vi "Measurement UI.vi"() -> ()   [LabVIEW 2021, in "Line Regulation_PMIC.lvlib"]
uses:
  Line Regulation_PMIC.lvlib
panel:
  in  "MeasGraphs":T1(tab)
  out "LineRegulationGraph(V/V)":T2(graph)
  out "LineRegulationGraph(%)":T3(graph)
  out "Load voltage deviation":dbl[](array[numeric])
  out "Load voltages":dbl[](array[numeric])
  out "Source voltages":dbl[](array[numeric])
  in  "Source resource name":string caption="RESOURCE NAME"
  in  "Load resource name":string caption="RESOURCE NAME"
  out "Measured current limit":dbl format="%#_6p"
  out "Measured voltage level":dbl format="%#_6p"
  out "Status":string
  in  "ELOADResourceName":refnum<k15> caption="RESOURCE NAME"
  in  "PPSResourceName":refnum<k15> caption="RESOURCE NAME"
  in  "Source sweep type":string(combo)="Logarithmic" caption="SWEEP TYPE"
  in  "DUT setup time":dbl=1.0 caption="DUT SETUP TIME" format="%#_6ps"
  in  "Source stop voltage":dbl=20.0 caption="STOP VOLTAGE" format="%#_6pV"
  in  "Source start voltage":dbl=6.0 caption="START VOLTAGE" format="%#_6pV"
  in  "Source voltage sweep points/points per decade":i32=10 caption="PTS/PTS PER DECADE"
  in  "Aperture time":dbl=0.005 caption="APERTURE TIME" format="%#_6ps"
  in  "Source delay":dbl=0.005 caption="SOURCE DELAY" format="%#_6ps"
  in  "Load current level":dbl=1.0 caption="CURRENT  LEVEL" format="%#_6pA"
  in  "Load voltage limit range":dbl=6.0 caption="VOLTAGE LIMIT RANGE" format="%#_6pV"
  in  "Source current limit":dbl=25.0 caption="CURRENT LIMIT" format="%#_6pA"
  in  "Source maximum power":dbl=300.0 caption="MAXIMUM POWER" format="%#_6pW"
  in  "Load configuration":string="Load configuration"
  in  "Source configuration":string="Source configuration"
  in  "Measurement settings":string="Measurement settings"
  in  "Nominal output voltage":dbl=3.3 caption="NOMINAL OUTPUT VOLTAGE" format="%#_6pV"
  in  "Mode of operation":T4(ring)=enum."Perform measurement" caption="MODE OF OPERATION"
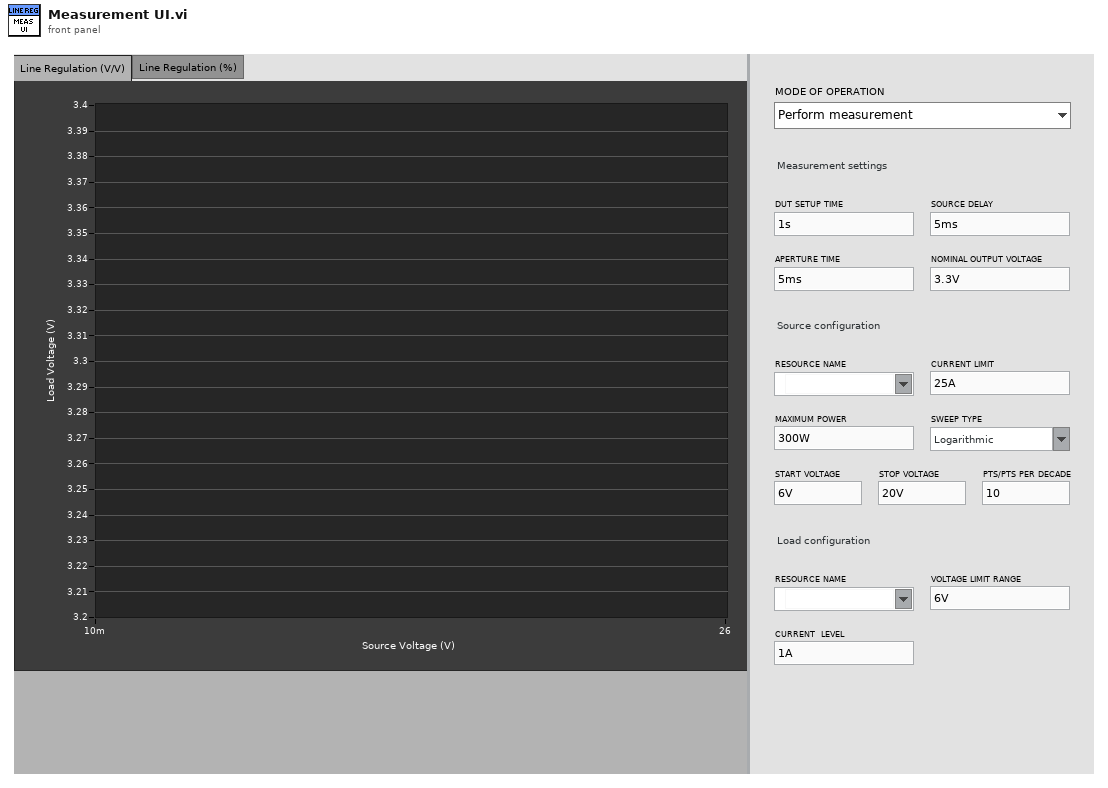
[diagram p1: front panel]
types:
  T1 = enum32{"Line Regulation (V/V)", "Line Regulation (%)", "Hidden Controls"}
  T2 = cluster{"Source voltages":dbl[], "Load voltages":dbl[]}
  T3 = cluster{"Source voltages":dbl[], "Load voltage deviation":dbl[]}
  T4 = enum32{"Power on the DUT", "Perform measurement", "Power off the DUT"}
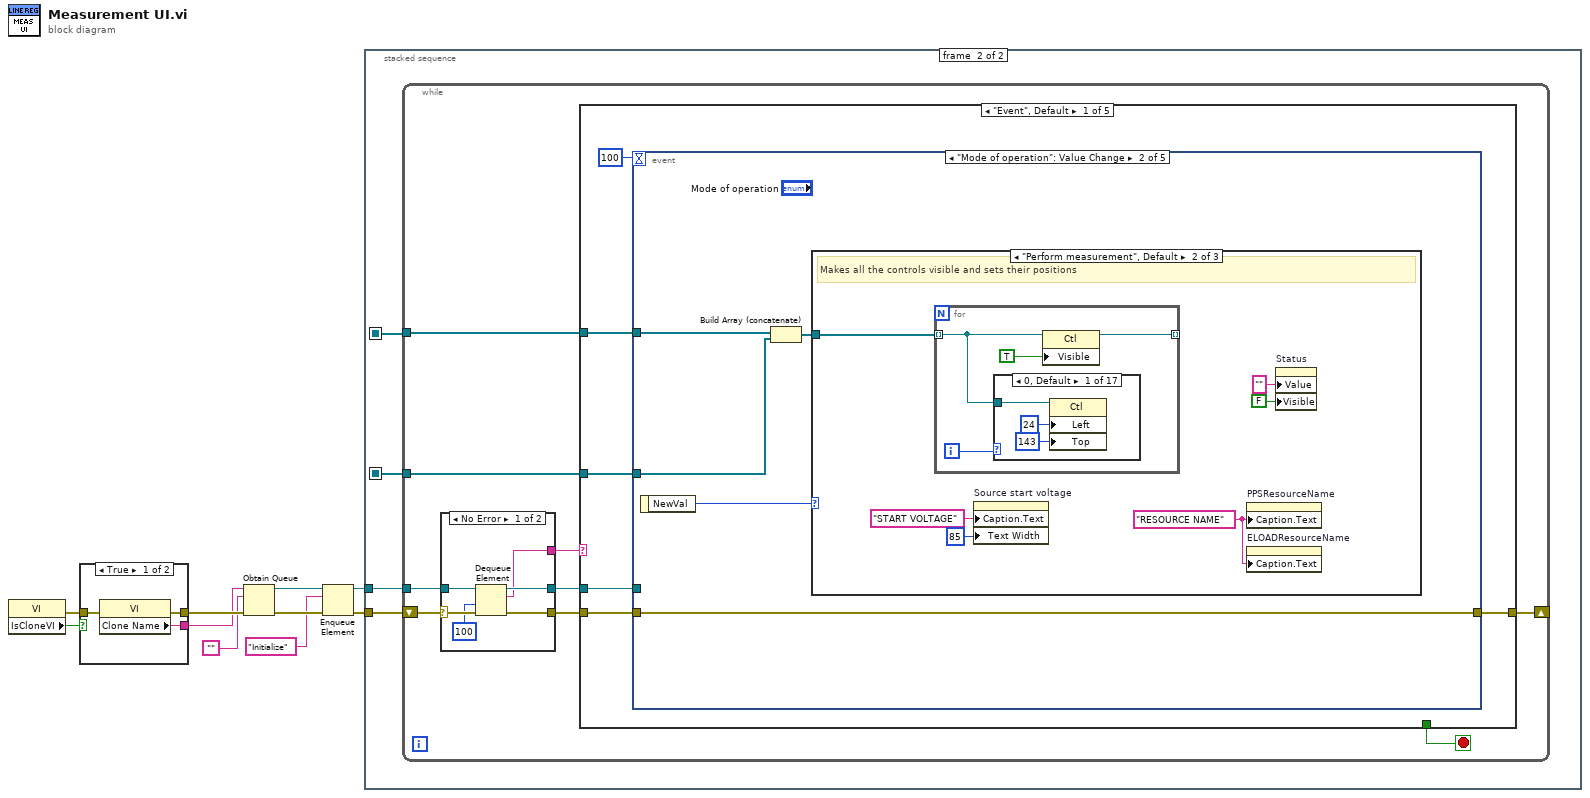
[diagram p0: block diagram]
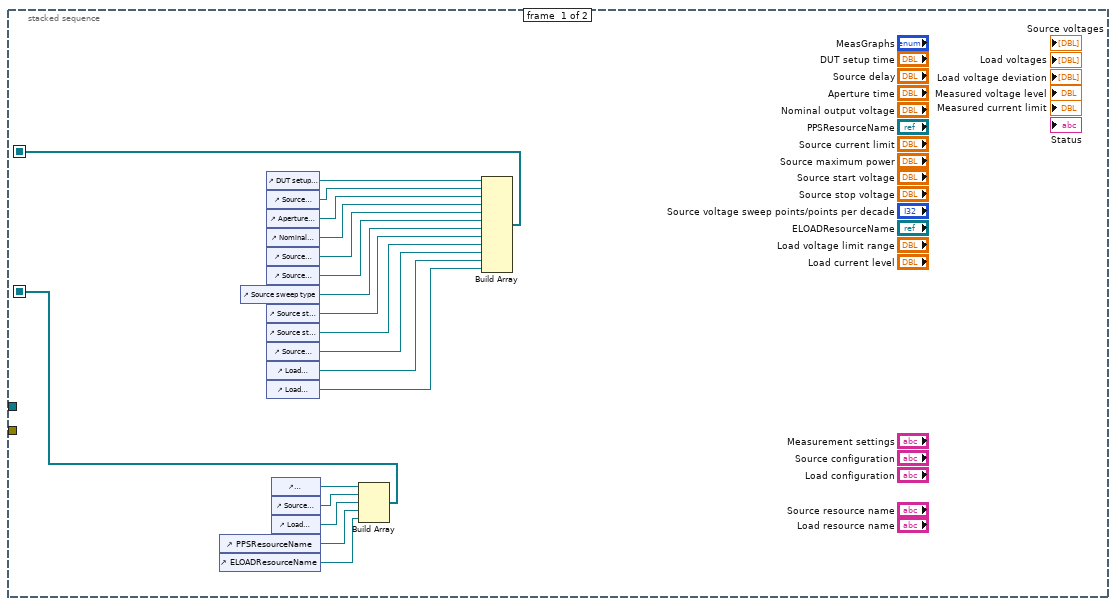
[diagram p2: hidden frame]
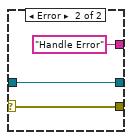
[diagram p3: hidden frame]
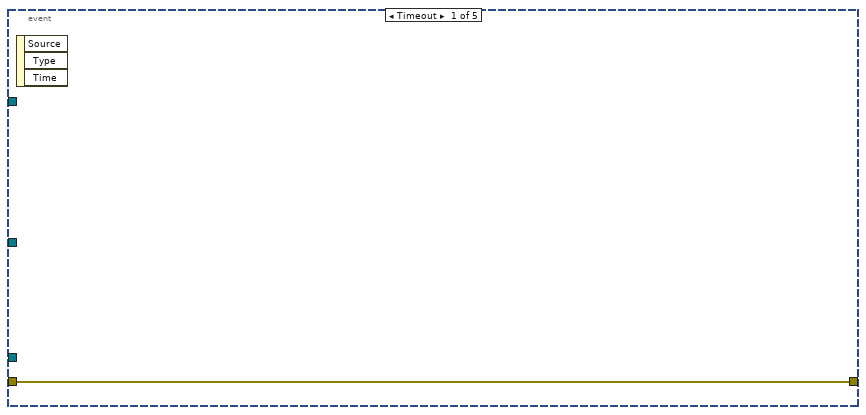
[diagram p4: hidden frame]
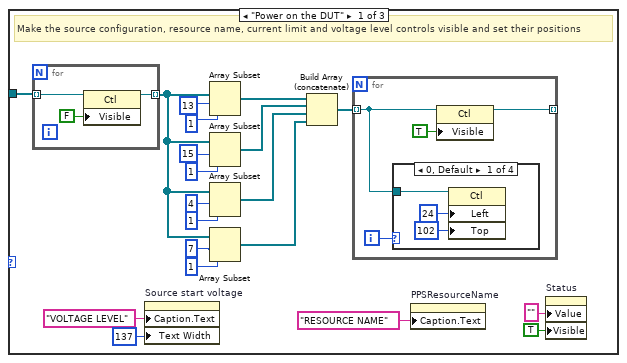
[diagram p5: hidden frame]
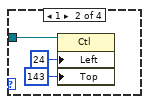
[diagram p6: hidden frame]
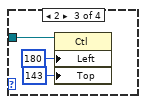
[diagram p7: hidden frame]
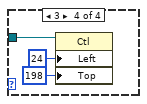
[diagram p8: hidden frame]
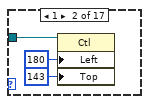
[diagram p9: hidden frame]
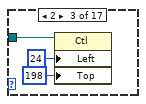
[diagram p10: hidden frame]
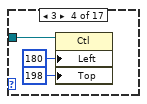
[diagram p11: hidden frame]
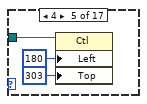
[diagram p12: hidden frame]
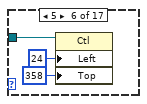
[diagram p13: hidden frame]
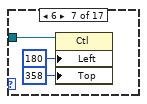
[diagram p14: hidden frame]
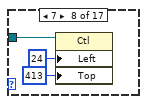
[diagram p15: hidden frame]
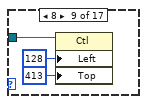
[diagram p16: hidden frame]
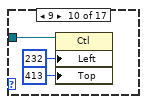
[diagram p17: hidden frame]
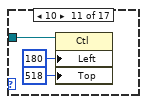
[diagram p18: hidden frame]
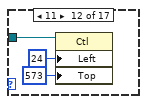
[diagram p19: hidden frame]
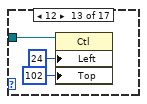
[diagram p20: hidden frame]
diagram:
  n1 = property class="VI"() -> (error out=w1:errorcluster, "IsCloneVI"=w2:bool)  [unwired: 2 in, 1 out]
  n2 = case shown="True" w2 {
    tunnel: [w13 w16] -> w10
    tunnel: [w12 w15] -> w9
    tunnel: w1 -> [w11 w14]
    frame True {
      n3 = property class="VI"(error in=w11) -> (error out=w13:errorcluster, "Clone Name"=w12:string)  [unwired: 1 in, 1 out]
    }
    frame False {
      n4 = property class="VI"(error in=w14) -> (error out=w16:errorcluster, "Name"=w15:string)  [unwired: 1 in, 1 out]
    }
  }
  n5 = Obtain Queue(name (unnamed)=w9, element data type="", error in (no error)=w10) -> (queue out=w6:refnum<queue>, error out=w8:errorcluster)  [unwired: 2 in, 1 out]
  n6 = Enqueue Element(queue=w6, element="Initialize", error in (no error)=w8) -> (queue out=w5:refnum<queue>, error out=w7:errorcluster)  [unwired: 1 in, 1 out]
  n7 = stacked-sequence {
    seq-local: [w18 _] -> [_ w37]
    seq-local: [w17 _] -> [_ w36]
    tunnel: w7 -> [_ w39]
    tunnel: w5 -> [_ w38]
    frame #0 {
      n8 = control-ref of="PPSResourceName"() -> (w21:refnum<vi>)
      n9 = control-ref of="ELOADResourceName"() -> (w20:refnum<vi>)
      n10 = control-ref of="Source sweep type"() -> (w19:refnum<vi>)
      n11 = control-ref of="DUT setup time"() -> (w35:refnum<vi>)
      n12 = control-ref of="Source delay"() -> (w34:refnum<vi>)
      n13 = control-ref of="Aperture time"() -> (w33:refnum<vi>)
      n14 = control-ref of="Nominal output voltage"() -> (w25:refnum<vi>)
      n15 = control-ref of="Source current limit"() -> (w32:refnum<vi>)
      n16 = control-ref of="Source maximum power"() -> (w31:refnum<vi>)
      n17 = control-ref of="Source start voltage"() -> (w30:refnum<vi>)
      n18 = control-ref of="Source stop voltage"() -> (w29:refnum<vi>)
      n19 = control-ref of="Source voltage sweep points/points per decade"() -> (w28:refnum<vi>)
      n20 = control-ref of="Load voltage limit range"() -> (w27:refnum<vi>)
      n21 = control-ref of="Load current level"() -> (w26:refnum<vi>)
      n22 = control-ref of="Measurement settings"() -> (w24:refnum<vi>)
      n23 = control-ref of="Source configuration"() -> (w22:refnum<vi>)
      n24 = control-ref of="Load configuration"() -> (w23:refnum<vi>)
      n25 = Build Array(w24, w22, w23, w21, w20) -> (w17:refnum<vi>[])
      n26 = Build Array(w35, w34, w33, w25, w32, w31, w19, w30, w29, w28, w27, w26) -> (w18:refnum<vi>[])
    }
    frame #1 {
      n27 = while {
        shift-right: [w43] -> _
        shift-left: w39 -> [w48]
        tunnel: w38 -> [w46]
        tunnel: w37 -> [w41]
        tunnel: w36 -> [w40]
        stop <- w42 stop-if-true
        n28 = case shown="No Error" w48 {
          selector: w48 -> [w54 w57]
          tunnel: [w53 w57] -> w47
          tunnel: w46 -> [w52 w56]
          tunnel: [w51 w56] -> w45
          tunnel: [w50 "Handle Error"] -> w44
          frame No Error {
            n29 = Dequeue Element(queue=w52, timeout in ms (-1)=100, error in (no error)=w54) -> (queue out=w51:refnum<queue>, element=w50:string, error out=w53:errorcluster)  [unwired: 1 out]
          }
          frame Error {
          }
        }
        n30 = case shown="\"Event\", Default" w44 {
          tunnel: w47 -> [w62 w206 w221 w235 w236]
          tunnel: w45 -> [w60 _ _ w233 _]
          tunnel: [w63 w206 w221 w227 w236] -> w43
          tunnel: [_ _ _ TRUE _] -> w42
          tunnel: w41 -> [w59 _ _ w226 _]
          tunnel: w40 -> [w58 _ _ w225 _]
          frame "Event", Default {
            n31 = event shown="[1] \"Mode of operation\": Value Change" {
              selector: _ -> [_ _ _ _ _]
              dyn-events: _ -> [_ _ _ _ _]
              timeout: 100 -> [_ _ _ _ _]
              tunnel: [w64 w65 w192 w194 w198] -> w63
              tunnel: w62 -> [w64 w65 w192 w194 w199]
              tunnel: w60 -> [_ _ _ _ w197]
              tunnel: w59 -> [_ w66 _ _ _]
              tunnel: w58 -> [_ w68 _ _ _]
              event Timeout {
                n32 = event-data() -> ()  [unwired: 1 in, 3 out]
              }
              event "Mode of operation": Value Change {
                n33 = event-data() -> ("NewVal"=w69:T4)  [unwired: 1 in]
                n34 = Build Array (concatenate)(w66, w68) -> (w67:refnum<vi>[])
                n35 = case shown="\"Perform measurement\", Default" w69 {
                  tunnel: w67 -> [w81 w114 w175]
                  frame "Power on the DUT" {
                    # "Make the source configuration, resource name, current limit and voltage level controls visible and set their positions"
                    n36 = for {
                      tunnel: w81 -> [w92] mode=indexing
                      tunnel: [w90] -> w78 mode=indexing
                      n37 = property class="Ctl"(reference=w92, "Visible"=FALSE) -> (reference out=w90:refnum<vi>)  [unwired: 1 in, 1 out]
                    }
                    n38 = property on="Source start voltage" class="DigNum (strict)"("Caption.Text"="VOLTAGE LEVEL", "Text Width"=u32 137) -> ()  [unwired: 2 in, 2 out]
                    n39 = Array Subset(array=w78, index=13 ("length"), length=1 ("index")) -> (w80:refnum<vi>[])
                    n40 = Array Subset(array=w78, index=15 ("length"), length=1 ("index")) -> (w79:refnum<vi>[])
                    n41 = Array Subset(array=w78, index=4 ("length"), length=1 ("index")) -> (w77:refnum<vi>[])
                    n42 = Array Subset(array=w78, index=7 ("length"), length=1 ("index")) -> (w75:refnum<vi>[])
                    n43 = Build Array (concatenate)(w80, w79, w77, w75) -> (w76:refnum<vi>[])
                    n44 = for {
                      tunnel: [w95] -> _ mode=indexing
                      tunnel: w76 -> [w93] mode=indexing
                      i -> [w94]
                      n45 = case shown="0, Default" w94 {
                        tunnel: w93 -> [w99 w102 w105 w108]
                        frame 0, Default {
                          n46 = property class="Ctl"(reference=w99, "Left"=24 ("Position:Left"), "Top"=102 ("Position:Top")) -> ()  [unwired: 1 in, 2 out]
                        }
                        frame 1 {
                          n47 = property class="Ctl"(reference=w102, "Left"=24 ("Position:Left"), "Top"=143 ("Position:Top")) -> ()  [unwired: 1 in, 2 out]
                        }
                        frame 2 {
                          n48 = property class="Ctl"(reference=w105, "Left"=180 ("Position:Left"), "Top"=143 ("Position:Top")) -> ()  [unwired: 1 in, 2 out]
                        }
                        frame 3 {
                          n49 = property class="Ctl"(reference=w108, "Left"=24 ("Position:Left"), "Top"=198 ("Position:Top")) -> ()  [unwired: 1 in, 2 out]
                        }
                      }
                      n50 = property class="Ctl"(reference=w93, "Visible"=TRUE) -> (reference out=w95:refnum<vi>)  [unwired: 1 in, 1 out]
                    }
                    n51 = property on="PPSResourceName" class="IVIName"("Caption.Text"="RESOURCE NAME") -> ()  [unwired: 2 in, 2 out]
                    n52 = property on="Status" class="Str"("Value"="" ("Operation"), "Visible"=TRUE) -> ()  [unwired: 2 in, 2 out]
                  }
                  frame "Perform measurement", Default {
                    w112 = "RESOURCE NAME" ("Caption.Text")
                    # "Makes all the controls visible and sets their positions"
                    n53 = for {
                      tunnel: w114 -> [w115] mode=indexing
                      tunnel: [w117] -> _ mode=indexing
                      i -> [w116]
                      n54 = case shown="0, Default" w116 {
                        tunnel: w115 -> [w121 w124 w127 w130 w133 w136 w139 w142 w145 w148 w151 w154 w157 w160 w163 w166 w169]
                        frame 0, Default {
                          n55 = property class="Ctl"(reference=w121, "Left"=24 ("Position:Left"), "Top"=143 ("Position:Top")) -> ()  [unwired: 1 in, 2 out]
                        }
                        frame 1 {
                          n56 = property class="Ctl"(reference=w124, "Left"=180 ("Position:Left"), "Top"=143 ("Position:Top")) -> ()  [unwired: 1 in, 2 out]
                        }
                        frame 2 {
                          n57 = property class="Ctl"(reference=w127, "Left"=24 ("Position:Left"), "Top"=198 ("Position:Top")) -> ()  [unwired: 1 in, 2 out]
                        }
                        frame 3 {
                          n58 = property class="Ctl"(reference=w130, "Left"=180 ("Position:Left"), "Top"=198 ("Position:Top")) -> ()  [unwired: 1 in, 2 out]
                        }
                        frame 4 {
                          n59 = property class="Ctl"(reference=w133, "Left"=180 ("Position:Left"), "Top"=303 ("Position:Top")) -> ()  [unwired: 1 in, 2 out]
                        }
                        frame 5 {
                          n60 = property class="Ctl"(reference=w136, "Left"=24 ("Position:Left"), "Top"=358 ("Position:Top")) -> ()  [unwired: 1 in, 2 out]
                        }
                        frame 6 {
                          n61 = property class="Ctl"(reference=w139, "Left"=180 ("Position:Left"), "Top"=358 ("Position:Top")) -> ()  [unwired: 1 in, 2 out]
                        }
                        frame 7 {
                          n62 = property class="Ctl"(reference=w142, "Left"=24 ("Position:Left"), "Top"=413 ("Position:Top")) -> ()  [unwired: 1 in, 2 out]
                        }
                        frame 8 {
                          n63 = property class="Ctl"(reference=w145, "Left"=128 ("Position:Left"), "Top"=413 ("Position:Top")) -> ()  [unwired: 1 in, 2 out]
                        }
                        frame 9 {
                          n64 = property class="Ctl"(reference=w148, "Left"=232 ("Position:Left"), "Top"=413 ("Position:Top")) -> ()  [unwired: 1 in, 2 out]
                        }
                        frame 10 {
                          n65 = property class="Ctl"(reference=w151, "Left"=180 ("Position:Left"), "Top"=518 ("Position:Top")) -> ()  [unwired: 1 in, 2 out]
                        }
                        frame 11 {
                          n66 = property class="Ctl"(reference=w154, "Left"=24 ("Position:Left"), "Top"=573 ("Position:Top")) -> ()  [unwired: 1 in, 2 out]
                        }
                        frame 12 {
                          n67 = property class="Ctl"(reference=w157, "Left"=24 ("Position:Left"), "Top"=102 ("Position:Top")) -> ()  [unwired: 1 in, 2 out]
                        }
                        frame 13 {
                          n68 = property class="Ctl"(reference=w160, "Left"=24 ("Position:Left"), "Top"=262 ("Position:Top")) -> ()  [unwired: 1 in, 2 out]
                        }
                        frame 14 {
                          n69 = property class="Ctl"(reference=w163, "Left"=24 ("Position:Left"), "Top"=477 ("Position:Top")) -> ()  [unwired: 1 in, 2 out]
                        }
                        frame 15 {
                          n70 = property class="Ctl"(reference=w166, "Left"=24 ("Position:Left"), "Top"=303 ("Position:Top")) -> ()  [unwired: 1 in, 2 out]
                        }
                        frame 16 {
                          n71 = property class="Ctl"(reference=w169, "Left"=24 ("Position:Left"), "Top"=518 ("Position:Top")) -> ()  [unwired: 1 in, 2 out]
                        }
                      }
                      n72 = property class="Ctl"(reference=w115, "Visible"=TRUE) -> (reference out=w117:refnum<vi>)  [unwired: 1 in, 1 out]
                    }
                    n73 = property on="Source start voltage" class="DigNum (strict)"("Caption.Text"="START VOLTAGE", "Text Width"=u32 85) -> ()  [unwired: 2 in, 2 out]
                    n74 = property on="PPSResourceName" class="IVIName"("Caption.Text"=w112) -> ()  [unwired: 2 in, 2 out]
                    n75 = property on="ELOADResourceName" class="IVIName"("Caption.Text"=w112) -> ()  [unwired: 2 in, 2 out]
                    n76 = property on="Status" class="Str"("Value"="" ("Status"), "Visible"=FALSE) -> ()  [unwired: 2 in, 2 out]
                  }
                  frame "Power off the DUT" {
                    # "Makes only the Source and Load Resource Name controls visible and sets their positions"
                    n77 = for {
                      tunnel: w175 -> [w180] mode=indexing
                      tunnel: [w179] -> w174 mode=indexing
                      n78 = property class="Ctl"(reference=w180, "Visible"=FALSE) -> (reference out=w179:refnum<vi>)  [unwired: 1 in, 1 out]
                    }
                    n79 = Array Subset(array=w174, index=15 ("length"), length=2 ("index")) -> (w176:refnum<vi>[])
                    n80 = property on="PPSResourceName" class="IVIName"("Caption.Text"="SOURCE RESOURCE NAME") -> ()  [unwired: 2 in, 2 out]
                    n81 = property on="ELOADResourceName" class="IVIName"("Caption.Text"="LOAD RESOURCE NAME") -> ()  [unwired: 2 in, 2 out]
                    n82 = for {
                      tunnel: w176 -> [w182] mode=indexing
                      tunnel: [w184] -> _ mode=indexing
                      i -> [w183]
                      n83 = case shown="0, Default" w183 {
                        tunnel: w182 -> [w188 w191]
                        frame 0, Default {
                          n84 = property class="Ctl"(reference=w188, "Left"=24 ("Position:Left"), "Top"=102 ("Position:Top")) -> ()  [unwired: 1 in, 2 out]
                        }
                        frame 1 {
                          n85 = property class="Ctl"(reference=w191, "Left"=24 ("Position:Left"), "Top"=157 ("Position:Top")) -> ()  [unwired: 1 in, 2 out]
                        }
                      }
                      n86 = property class="Ctl"(reference=w182, "Visible"=TRUE) -> (reference out=w184:refnum<vi>)  [unwired: 1 in, 1 out]
                    }
                    n87 = property on="Status" class="Str"("Value"="" ("Operation"), "Visible"=TRUE) -> ()  [unwired: 2 in, 2 out]
                  }
                }
              }
              event "PPSResourceName": Value Change {
                n88 = event-data() -> ()  [unwired: 1 in, 1 out]
                n89 = property on="PPSResourceName" class="IVIName"() -> ("Value"=w193:refnum<k15>)  [unwired: 2 in, 2 out]
                n90 = property on="Source resource name" class="Str"("Value"=w193) -> ()  [unwired: 2 in, 2 out]
              }
              event "ELOADResourceName": Value Change {
                n91 = event-data() -> ()  [unwired: 1 in, 1 out]
                n92 = property on="ELOADResourceName" class="IVIName"() -> ("Value"=w195:refnum<k15>)  [unwired: 2 in, 2 out]
                n93 = property on="Load resource name" class="Str"("Value"=w195) -> ()  [unwired: 2 in, 2 out]
              }
              event Panel Close? {
                n94 = event-data() -> ()  [unwired: 1 in, 1 out]
                n95 = Enqueue Element(queue=w197, element="Exit", error in (no error)=w199) -> (error out=w198:errorcluster)  [unwired: 1 in, 2 out]
                n96 = event-data("Discard?"=TRUE) -> ()  [unwired: 1 in, 1 out]
              }
            }
          }
          frame "Initialize" {
            w205 = "<Select Device>"
            n97 = control-ref of="LineRegulationGraph(V/V)"() -> (w204:refnum<vi>)
            n98 = control-ref of="LineRegulationGraph(%)"() -> (w203:refnum<vi>)
            n99 = Build Array(w204, w203) -> (w202:refnum<vi>[])
            n100 = for {
              tunnel: w202 -> [w207] mode=indexing
              n101 = property class="XYGraph (strict)"(reference=w207, "ActPaletteTool"=2 ("Palette:Active Tool")) -> ()  [unwired: 1 in, 2 out]
            }
            n102 = property on="PPSResourceName" class="IVIName"("Value"=w205) -> ()  [unwired: 2 in, 2 out]
            n103 = property on="ELOADResourceName" class="IVIName"("Value"=w205) -> ()  [unwired: 2 in, 2 out]
            n104 = property on="Status" class="Str"("Visible"=FALSE) -> ()  [unwired: 2 in, 2 out]
          }
          frame "Post UI Update" {
            # "This case will be triggered, after framework updates the User interface with result values."
            n105 = control-ref of="LineRegulationGraph(V/V)"() -> (w211:refnum<vi>)
            n106 = control-ref of="LineRegulationGraph(%)"() -> (w210:refnum<vi>)
            n107 = Not Equal?(x="Linear", y="Source sweep type") -> (x != y?=w214:bool)
            n108 = Build Array(w211, w210) -> (w209:refnum<vi>[])
            n109 = Boolean To (0,1)(Boolean=w214) -> (0, 1=w213:i16)
            n110 = for {
              tunnel: w209 -> [w223] mode=indexing
              tunnel: w213 -> [w222]
              n111 = property class="XYGraph (strict)"(reference=w223, "XScale.Mapping Mode"=w222) -> ()  [unwired: 1 in, 2 out]
            }
            n112 = local read "Load voltage deviation"() -> (w219:dbl[])
            n113 = local read "Source voltages"() -> (w218:dbl[])
            n114 = local read "Load voltages"() -> (w220:dbl[])
            n115 = Bundle("Source voltages"=w218, "Load voltages"=w220) -> (→"LineRegulationGraph(V/V)":T2)  [unwired: 1 in]
            n116 = Bundle("Source voltages"=w218, "Load voltage deviation"=w219) -> (→"LineRegulationGraph(%)":T3)  [unwired: 1 in]
          }
          frame "Exit" {
            # "This case is triggered to close the User Interface from framework"
            n117 = Build Array (concatenate)(w226, w225) -> (w224:refnum<vi>[])
            n118 = Close Reference(reference=w224) -> (error out=w229:errorcluster)  [unwired: 1 in]
            n119 = Flush Queue(queue=w233, error in (no error)=w235) -> (queue out=w232:refnum<queue>, error out=w231:errorcluster)  [unwired: 1 out]
            n120 = Release Queue(queue=w232, force destroy? (F)=TRUE, error in (no error)=w231) -> (error out=w228:errorcluster)  [unwired: 2 out]
            n121 = Merge Errors(w229, w228) -> (w227:errorcluster)
          }
          frame "Handle Error" {
          }
        }
      }
    }
  }
